vi "RichToFlatrfcontrol_AuroraChangeStreamRequest.vi"(5 "OutputClusterType":T1, 11 "InputCluster":T2) -> (3 "OutputCluster":T1)   [LabVIEW 2024, in "FlexSDR_gRPC_client.lvlib"]
uses:
  FlexSDR_gRPC_client.lvlib
  rfcontrol_AuroraChangeStreamRequest.ctl
  rfcontrol_AuroraChangeStreamRequest_Flat.ctl
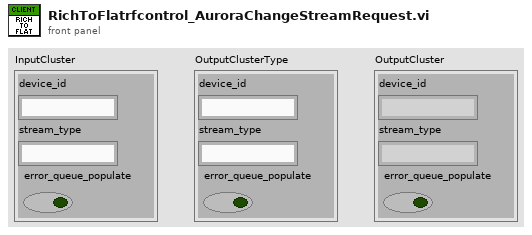
[diagram p1: front panel]
types:
  T1 = typedef "FlexSDR_gRPC_client.lvlib/rfcontrol_AuroraChangeStreamRequest_Flat.ctl" = cluster{"device_id":string, "stream_type":string, "error_queue_populate":bool}
  T2 = typedef "FlexSDR_gRPC_client.lvlib/rfcontrol_AuroraChangeStreamRequest.ctl" = cluster{"device_id":string, "stream_type":string, "error_queue_populate":bool}
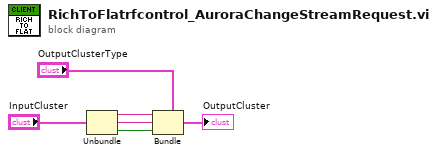
[diagram p0: block diagram]
diagram:
  n1 = Unbundle "Unbundle"("InputCluster") -> ("device_id"=w3:string, "stream_type"=w2:string, "error_queue_populate"=w1:bool)
  n2 = Bundle "Bundle"(cluster="OutputClusterType", "device_id"=w3, "stream_type"=w2, "error_queue_populate"=w1) -> (→"OutputCluster":T1)
